vi "dfd_Content String to Value.vi"(8 "error in (no error)":errorcluster, 11 "string":string) -> (0 "error out":errorcluster, 3 "value":dbl)   [LabVIEW 2017, in "NI_DigFilter_Process.lvlib"]
uses:
  <vilib>/addons/Digital Filter Design/NI_DigFilter_Process.lvlib
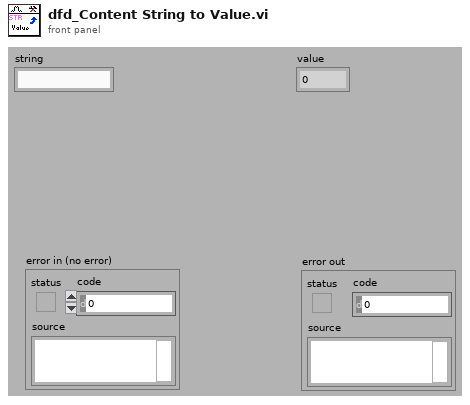
[diagram p1: front panel]
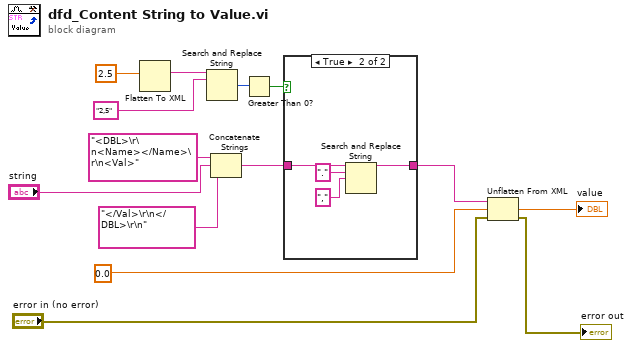
[diagram p0: block diagram]
diagram:
  n1 = Flatten To XML(anything=2.5) -> (xml string=w6:string)
  n2 = Search and Replace String(input string=w6, search string="2,5") -> (number of replacements=w4:i32)  [unwired: 1 in, 8 out]
  n3 = Concatenate Strings("<DBL>\r\n<Name></Name>\r\n<Val>", "string", "</Val>\r\n</DBL>\r\n") -> (w2:string)
  n4 = Greater Than 0?(x=w4) -> (x > 0?=w3:bool)
  n5 = case shown="True" w3 {
    tunnel: w2 -> [w15 w17]
    tunnel: [w15 w16] -> w1
    frame False {
    }
    frame True {
      n6 = Search and Replace String(input string=w17, search string=".", replace string="," ("replace string (\"\")")) -> (result string=w16:string)  [unwired: 2 in, 6 out]
    }
  }
  n7 = Unflatten From XML(xml string=w1, type=0.0 ("numeric"), error in (no error)="error in (no error)") -> (value=→"value":dbl, error out=→"error out":errorcluster)
